vi "DAQmx_CreateDigitalPuls.vi"(0 "lines":string[](array[string])=["Dev1/port0/line0"], 5 "data":u32[][](array[numeric]), 7 "rate":dbl=1000000.0, 11 "error in":errorcluster) -> (4 "task out":refnum<k21>, 15 "error out":errorcluster)   [LabVIEW 2010]
uses:
  <vilib>/DAQmx/write.llb/DAQmx Write.vi
  <vilib>/DAQmx/write.llb/DAQmx Write (Digital 2D U32 NChan NSamp).vi
  <vilib>/DAQmx/configure/timing.llb/DAQmx Timing (Sample Clock).vi
  <vilib>/DAQmx/configure/trigger.llb/DAQmx Trigger.vi
  <vilib>/DAQmx/configure/trigger.llb/DAQmx Start Trigger (Digital Edge).vi
  <vilib>/DAQmx/create/channels.llb/DAQmx Create Channel (DO-Digital Output).vi
  <vilib>/daqmx/miscellaneous.llb/DAQmx Fill In Error Info.vi
  Program Files/National Instruments/LabVIEW 2010/resource/objmgr/daqmx.rc
panel:
  in  "timeout (s)":dbl=10.0 format="%0.2f"
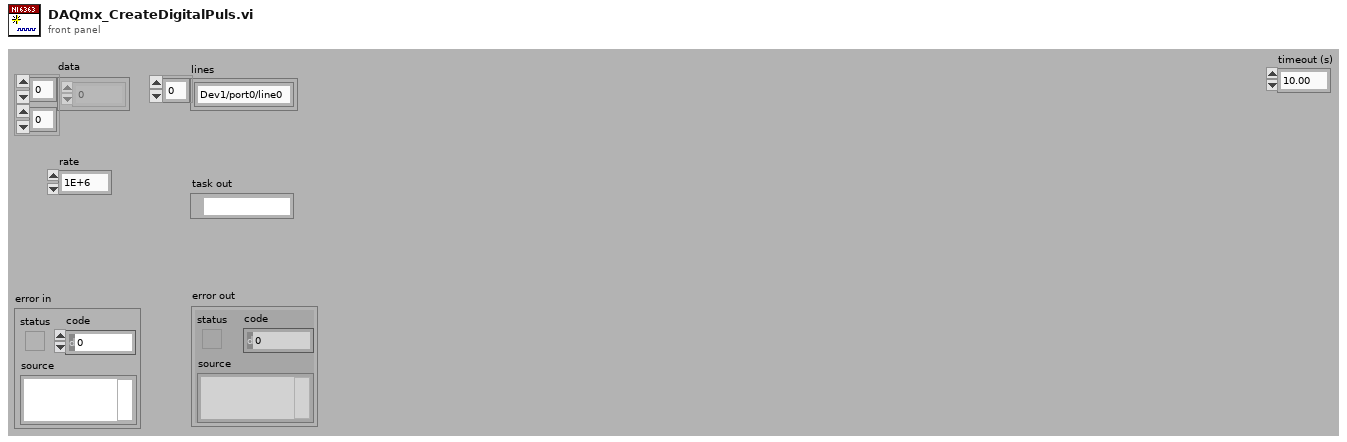
[diagram p1: front panel]
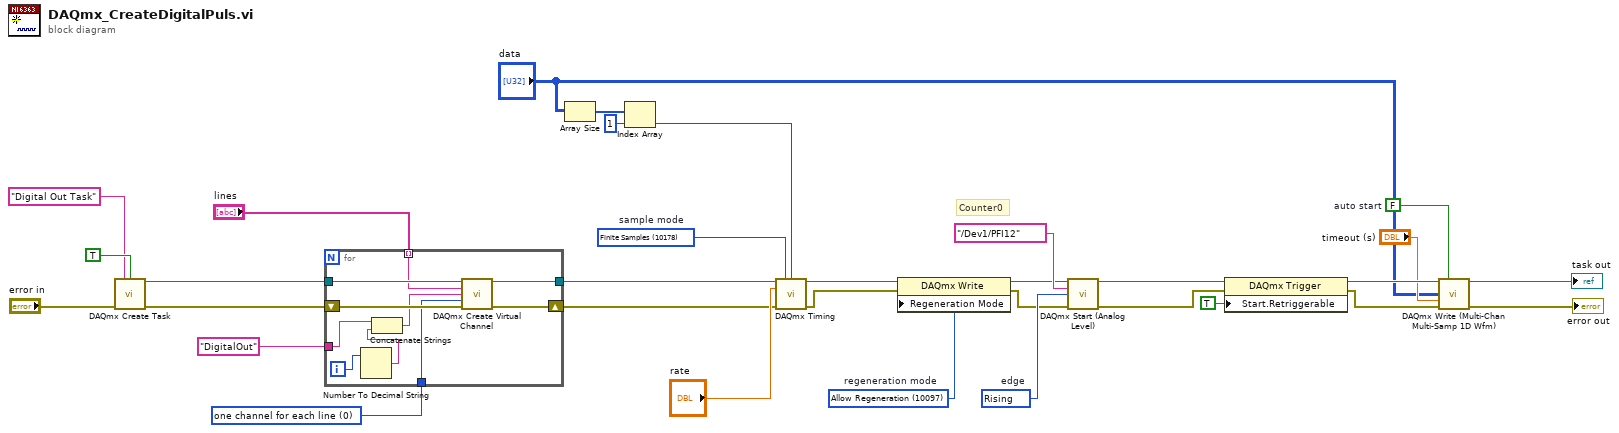
[diagram p0: block diagram]
diagram:
  w6 = 0 items=["one channel for each line", "one channel for all lines"] ("line grouping")
  w12 = FALSE  # auto start
  w21 = 10280 items=["Rising"=10280, "Falling"=10171]  # edge
  w24 = 10097 items=["Allow Regeneration"=10097, "Do Not Allow Regeneration"=10158]  # regeneration mode
  w27 = 10178 items=["Finite Samples"=10178, "Continuous Samples"=10123, "Hardware Timed Single Point"=12522]  # sample mode
  # "Counter0"
  n1 = call <vilib>:"DAQmx Create Task.vi"("new task name"="Digital Out Task", "auto cleanup"=TRUE, "error in"="error in") -> ("task out"=w29:refnum<k21>, "error out"=w30:errorcluster)  [unwired: 11 in]
  n2 = for {
    tunnel: w29 -> [w42]
    tunnel: [w40] -> w25
    tunnel: "lines" -> [w38] mode=indexing
    tunnel: "DigitalOut" ("channel name") -> [w35]
    tunnel: w6 -> [w37]
    shift-right: [w39] -> w26
    shift-left: w30 -> [w41]
    i -> [w36]
    n3 = Number To Decimal String(number=w36) -> (decimal integer string=w34:string)  [unwired: 1 in]
    n4 = Concatenate Strings(w35, w34) -> (w33:string)
    n5 = call-poly <vilib>:"DAQmx Create Virtual Channel.vi"("task in"=w42, "lines"=w38, "name to assign"=w33, "line grouping"=w37, "error in"=w41) -> ("task out"=w40:refnum<k21>, "error out"=w39:errorcluster)  [unwired: 9 in]
  }
  n6 = Array Size(array="data") -> (size(s)=w4:i32[])
  n7 = Index Array(array=w4, index=1) -> (element=w2:i32)
  n8 = call-poly <vilib>:"DAQmx Timing.vi"("task/channels in"=w25, "sample mode"=w27, "samples per channel"=w2, "rate"="rate", "error in"=w26) -> ("task out"=w22:refnum<k21>, "error out"=w23:errorcluster)  [unwired: 9 in]
  n9 = property class="DAQmx Write"(reference=w22, error in=w23, "Regeneration Mode"=w24) -> (reference out=w16:refnum<k21>, error out=w15:errorcluster)
  n10 = call-poly "DAQmx Start (Analog Level).vi"("task/channels in"=w16, "source"=tag "/Dev1/PFI12", "edge"=w21, "error in"=w15) -> ("task out"=w20:refnum<k21>, "error out"=w19:errorcluster)  [unwired: 10 in]
  n11 = property class="DAQmx Trigger"(reference=w20, error in=w19, "Start.Retriggerable"=TRUE) -> (reference out=w14:refnum<k21>, error out=w13:errorcluster)
  n12 = call-poly "DAQmx Write (Multi-Chan Multi-Samp 1D Wfm).vi"("task/channels in"=w14, "auto start"=w12, "data"="data", "timeout"="timeout (s)", "error in"=w13) -> ("task out"=→"task out":refnum<k21>, "error out"=→"error out":errorcluster)  [unwired: 8 in, 1 out]
